vi "TCP-IP Q_Bridge.Read Msg with Length Header.vi"(8 "error in (no error)":errorcluster, 9 "Timeoutms":i32=100, 11 "ConID":refnum<k5>) -> (0 "Error Out":errorcluster, 1 "Timed Out":bool, 2 "data out":string, 3 "ConID Out":refnum<k5>)   [LabVIEW 2024, in "EQMF.lvlib" / "TCP-IP.lvlib"]
uses:
  TCP-IP.lvlib
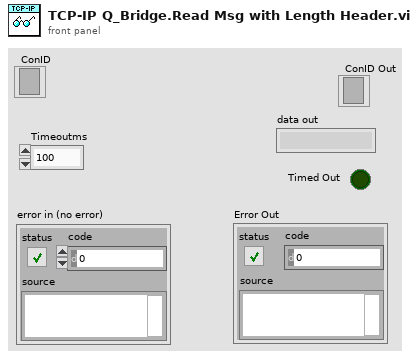
[diagram p1: front panel]
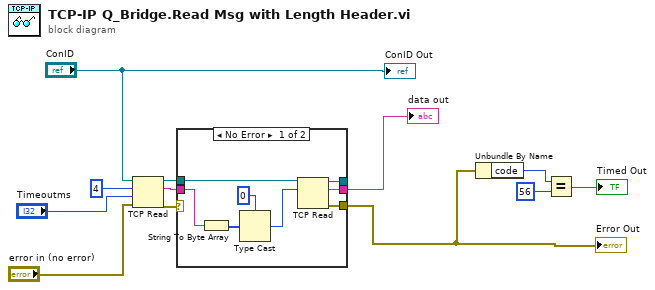
[diagram p0: block diagram]
diagram:
  n1 = TCP Read(connection ID="ConID", bytes to read=4, error in (no error)="error in (no error)", 9:"Timeoutms") -> (connection ID out=w9:refnum<k5>, data out=w11:string, error out=w10:errorcluster)  [unwired: 1 in]
  n2 = case shown="No Error" w10 {
    selector: w10 -> [_ w22]
    tunnel: w11 -> [w20 _]
    tunnel: w9 -> [w16 w21]
    tunnel: [w15 w21] -> _
    tunnel: [w14 _] -> w7
    tunnel: [w13 w22] -> w1
    frame No Error {
      n3 = String To Byte Array(string=w20) -> (unsigned byte array=w19:u8[])
      n4 = Type Cast(type=0, x=w19) -> (*(type *) &x=w17:i32)
      n5 = TCP Read(connection ID=w16, bytes to read=w17) -> (connection ID out=w15:refnum<k5>, data out=w14:string, error out=w13:errorcluster)  [unwired: 3 in]
    }
    frame Error {
    }
  }
  "Error Out" <- w1
  "data out" <- w7
  n6 = Unbundle By Name(w1) -> ("code"=w4:i32)
  n7 = Equal?(x=w4, y=56) -> (x = y?=→"Timed Out":bool)
  "ConID Out" <- "ConID"
